vi "Read data HW.vi"(8 "error in":errorcluster, 11 "HW Resource in":T1) -> (0 "error out":errorcluster, 2 "data":dbl[](array[numeric]) format="%0.2f", 3 "HW Resource out":T1)   [LabVIEW 2017, in "Acquisition.lvlib"]
uses:
  Acquisition.lvlib
  Control/Config chanel.ctl
  <vilib>/DAQmx/read.llb/DAQmx Read (Analog 1D DBL NChan 1Samp).vi
  <vilib>/DAQmx/miscellaneous.llb/DAQmx Fill In Error Info.vi
  <resource>/objmgr/daqmx.rc
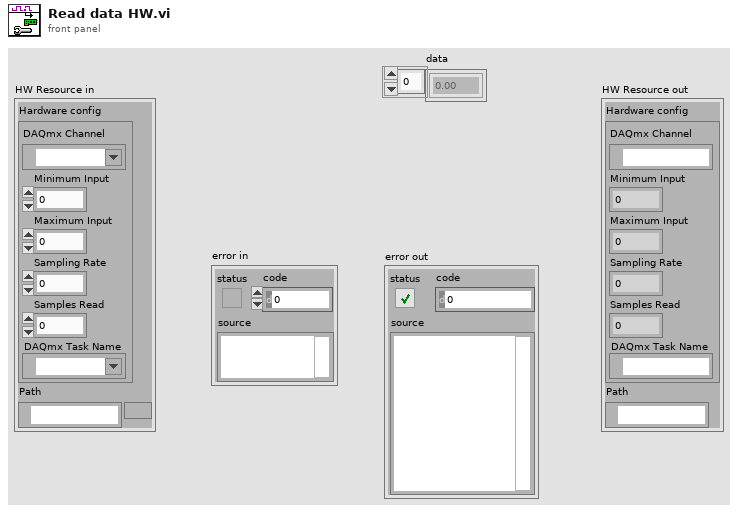
[diagram p1: front panel]
types:
  T1 = typedef "Config chanel.ctl" = cluster{"Hardware config":cluster{"DAQmx Channel":tag, "Minimum Input":dbl, "Maximum Input":dbl, "Sampling Rate":dbl, "Samples Read":dbl, "DAQmx Task Name":refnum<k21>}, "Path":path}
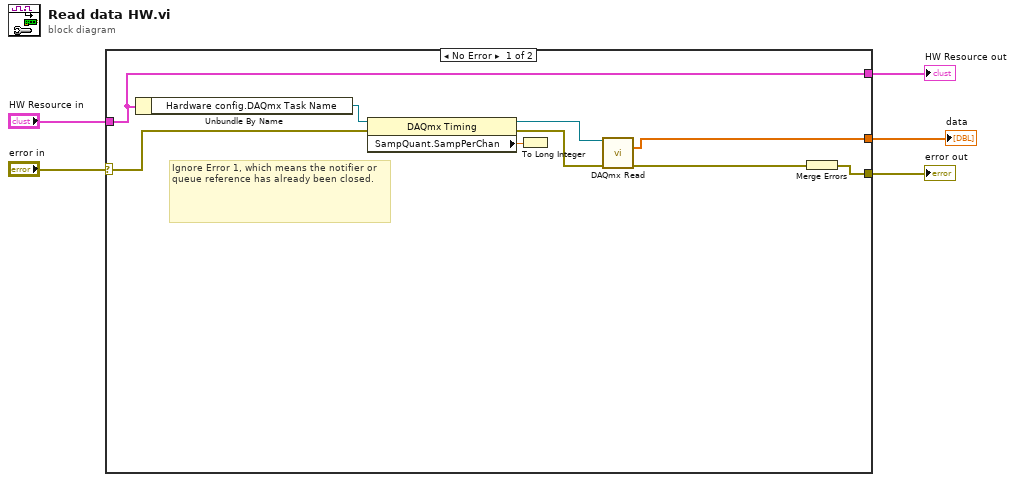
[diagram p0: block diagram]
diagram:
  n1 = case shown="No Error" "error in" {
    selector: "error in" -> [w10 w16]
    tunnel: "HW Resource in" -> [w14 w15]
    tunnel: [w7 w16] -> w3
    tunnel: [w14 w15] -> w2
    tunnel: [w6 _] -> w1
    frame No Error {
      # "Ignore Error 1, which means the notifier or queue reference has already been closed."
      n2 = Unbundle By Name(w14) -> ("Hardware config.DAQmx Task Name"=w13:refnum<k21>)
      n3 = property class="DAQmx Timing"(reference=w13, error in=w10) -> (reference out=w12:refnum<k21>, error out=w9:errorcluster, "SampQuant.SampPerChan"=w11:dbl)
      n4 = To Long Integer(number=w11) -> ()  [unwired: 1 out]
      n5 = call-poly <vilib>:"DAQmx Read.vi"("task/channels in"=w12, "error in"=w9) -> ("data"=w6:dbl[], "error out"=w8:errorcluster)  [unwired: 11 in, 1 out]
      n6 = Merge Errors(w8) -> (w7:errorcluster)
    }
    frame Error {
    }
  }
  "error out" <- w3
  "HW Resource out" <- w2
  "data" <- w1
